vi "TEST - Get Physical Units.vi"(8 "error in (no error)":errorcluster) -> (0 "error out":errorcluster, 2 "pass":bool)   [LabVIEW 2013]
uses:
  source/library/Physical Units.ctl
panel:
  out "Failures":T2(array[cluster])
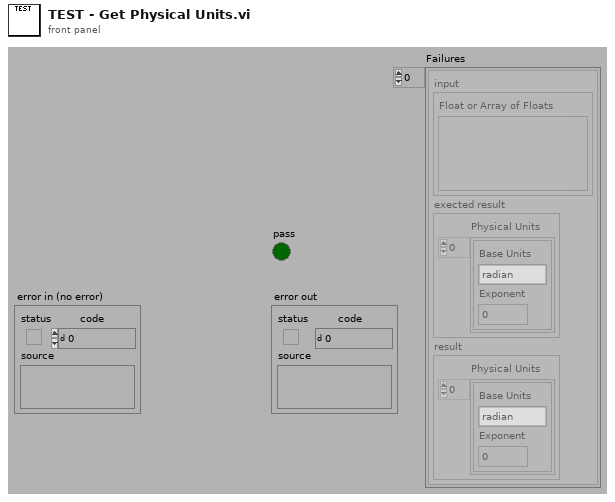
[diagram p1: front panel]
types:
  T1 = typedef "Physical Units.ctl" = cluster{"Base Units":enum16{"radian", "steradian", "second", "meter", "kilogram", "ampere", "kelvin", "mole", "candela"}, "Exponent":i16}
  T2 = cluster{"input":cluster{"Float or Array of Floats":variant}, "exected result":cluster{"Physical Units":T1[]}, "result":cluster{"Physical Units":T1[]}}[]
  T3 = cluster{"input":cluster{"Float or Array of Floats":variant}, "exected result":cluster{"Physical Units":T1[]}, "result":cluster{"Physical Units":T1[]}}
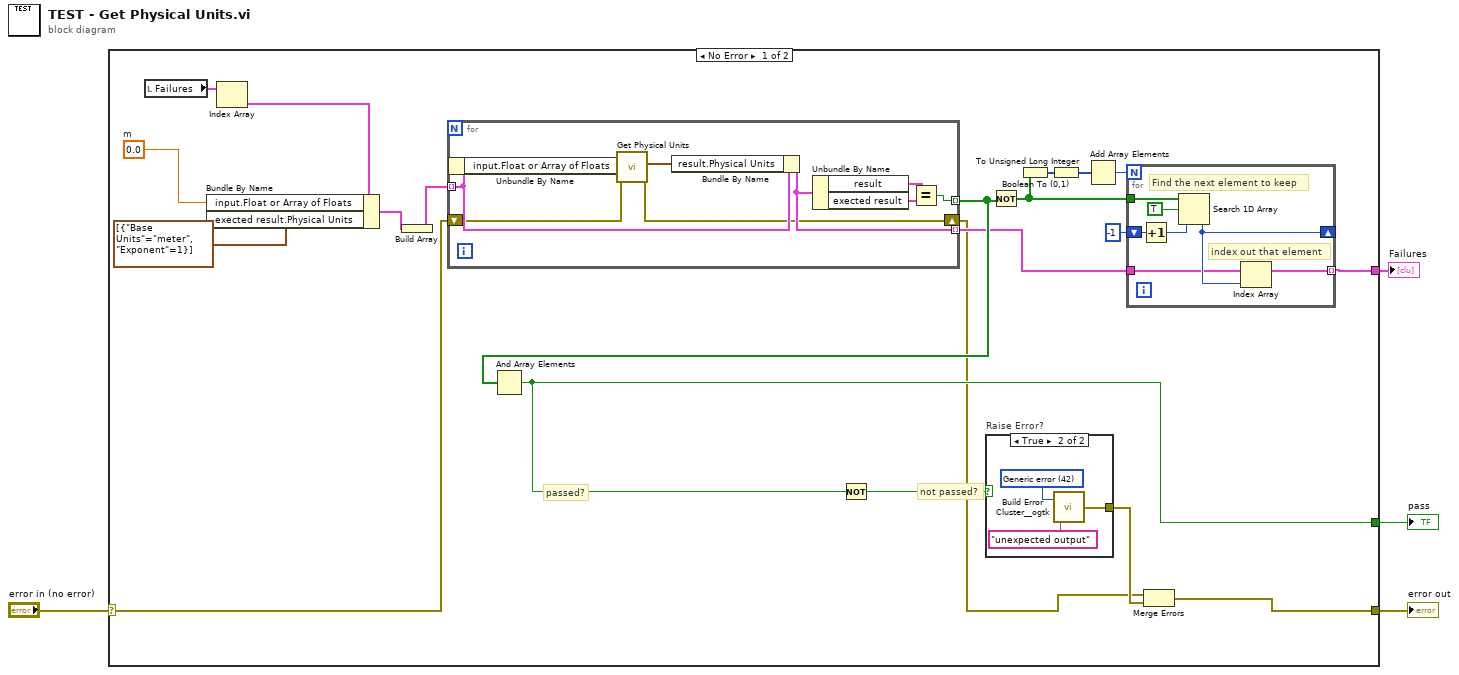
[diagram p0: block diagram]
diagram:
  n1 = case shown="No Error" "error in (no error)" {
    selector: "error in (no error)" -> [w10 w44]
    tunnel: [w21 _] -> w4
    tunnel: [w24 w44] -> w2
    tunnel: [w13 _] -> w1
    frame No Error {
      w5 = dbl[unit] 0.0  # m
      # "not passed?"
      # "passed?"
      n2 = local read "Failures"() -> (w8:T2)
      n3 = Index Array(array=w8) -> (element=w7:T3)  [unwired: 1 in]
      n4 = Bundle By Name(cluster=w7, "input.Float or Array of Floats"=w5, "exected result.Physical Units"=T1[] [{"Base Units"=enum."meter", "Exponent"=1}] ("Physical Units")) -> (w12:T3)
      n5 = Build Array(w12) -> (w11:T2)
      n6 = for {
        tunnel: w11 -> [w39] mode=indexing
        tunnel: [w40] -> w15 mode=indexing
        tunnel: [w38] -> w14 mode=indexing
        shift-right: [w33] -> w9
        shift-left: w10 -> [w32]
        n7 = Unbundle By Name(w39) -> ("input.Float or Array of Floats"=w35:variant)
        n8 = call "Get Physical Units.vi"("error in (no error)"=w32, "Float or Array of Floats"=w35) -> ("error out"=w33:errorcluster, "Physical Units"=w34:T1[])  [unwired: 8 in]
        n9 = Bundle By Name(cluster=w39, "result.Physical Units"=w34) -> (w38:T3)
        n10 = Unbundle By Name(w38) -> ("result"=w37:cluster{"Physical Units":T1[]}, "exected result"=w36:cluster{"Physical Units":T1[]})
        n11 = Equal?(x=w37, y=w36) -> (x = y?=w40:bool)
      }
      n12 = And Array Elements(Boolean array=w15) -> (logical AND=w21:bool)
      n13 = Not(x=w21) -> (.not. x?=w22:bool)
      n14 = case "Raise Error?" shown="True" w22 {
        tunnel: [_ w41] -> w23
        frame False {
        }
        frame True {
          w42 = 42 items=["No error", "Argument error", "Memory is full", "Out of zone", "End of file", "File already open", "Generic file I/O error", "File not found", "File permission error", "Disk is full", "Duplicate path", "Too many files open", "System feature not enabled", "Resource file not found", "Cannot add resource", "Resource not found", "Image not found", "Image memory error", "Pen does not exist", "Config type invalid", "Config token not found", "Config parse error", "Config memory error", "Bad external code format", "Bad external code offset", "External code not present", "Null window", "Destroy window error", "Null menu", "Print aborted", "Bad print record", "Print driver error", "Windows error during printing", "Memory error during printing", "Print dialog error", "Generic print error", "Invalid device refnum", "Device not found", "Device parameter error", "Device unit error", "Cannot open device", "Device call aborted", "Generic error", "Cancelled by user", "Object ID too low", "Object ID too high", "Object not in heap", "Unknown heap", "Unknown object (invalid DefProc)", "Unknown object (DefProc not in table)", "Message out of range", "Invalid (null) method", "Unknown message", "Manager call not supported", "Bad address", "Network operation in progress", "Network operation timed out", "Connection is busy", "Network attribute not supported", "Network error", "Address in use", "System out of memory", "Connection aborted", "Connection refused", "Not connected", "Already connected", "Connection closed", "Initialization error (interapplication manager)", "Bad occurrence", "Wait on unbound occurrence handler", "Occurrence queue overflow", "Datalog type conflict", "Unused", "Unrecognized type (interapplication manager)", "Memory corrupt", "Failed to make temporary DLL", "Old CIN version", "Drag socket not found", "Failed to load drop-object", "Failed to register OLE object", "Failed to release OLE object", "Format specifier type mismatch", "Unknown format specifier", "Too few format specifiers", "Too many format specifiers", "Scan failed", "Newer CIN version", "Error converting to variant", "Runtime menu error", "Password tampered", "Variant attribute not found", "Incompatible variant data type", "Event data is not available", "Event Store is not present", "Occurrence is not found", "Event Queue is not created", "Event info is not available", "Refnum passed is NULL", "Error retrieving Class GUID", "Error retrieving CoClass GUID", "Error retrieving TypeLib GUID.", "Bad built application magic bytes.", "Specific driver is different from the specific driver associated with the Logical Name.", "There is no session opened to the class driver.", "Max Error", "MAX - Error with config objects", "MAX - Error loading configuration", "MAX - Group not supported"]
          n15 = call <userlib>:"Build Error Cluster__ogtk.vi"("String to Prepend to source (\"\")"="unexpected output" ("String to Prepend to source (\"\")"), "code"=w42) -> ("error out"=w41:errorcluster)
        }
      }
      n16 = Not(x=w15) -> (.not. x?=w17:bool[])
      n17 = Boolean To (0,1)(Boolean=w17) -> (0, 1=w18:i16[])
      n18 = To Unsigned Long Integer(number=w18) -> (unsigned 32bit integer=w16:u32[])
      n19 = Add Array Elements(numeric array=w16) -> (sum=w19:u32)
      n20 = for {
        N: w19 -> [_]
        tunnel: w14 -> [w27]
        tunnel: w17 -> [w31]
        shift-right: [w28] -> _
        shift-left: -1 ("start index (0)") -> [w29]
        tunnel: [w26] -> w13 mode=indexing
        # "index out that element"
        # "Find the next element to keep"
        n21 = Increment(x=w29) -> (x+1=w25:i32)
        n22 = Search 1D Array(1D array=w31, element=TRUE, start index (0)=w25) -> (index of element=w28:i32)
        n23 = Index Array(array=w27, index=w28) -> (element=w26:T3)
      }
      n24 = Merge Errors(w9, w23) -> (w24:errorcluster)
    }
    frame Error {
    }
  }
  "pass" <- w4
  "error out" <- w2
  "Failures" <- w1
